vi "unregisterSubscriber.vi"(1 "Parameters":T2) -> (2 "Error out":errorcluster, 3 "Reply":T1, 4 "Reply":string, 5 "registerSubscriber":string)   [LabVIEW 2010]
uses:
  <userlib>/ROSforLV_0.1/ROS/Code/_ROSDefinition.vi
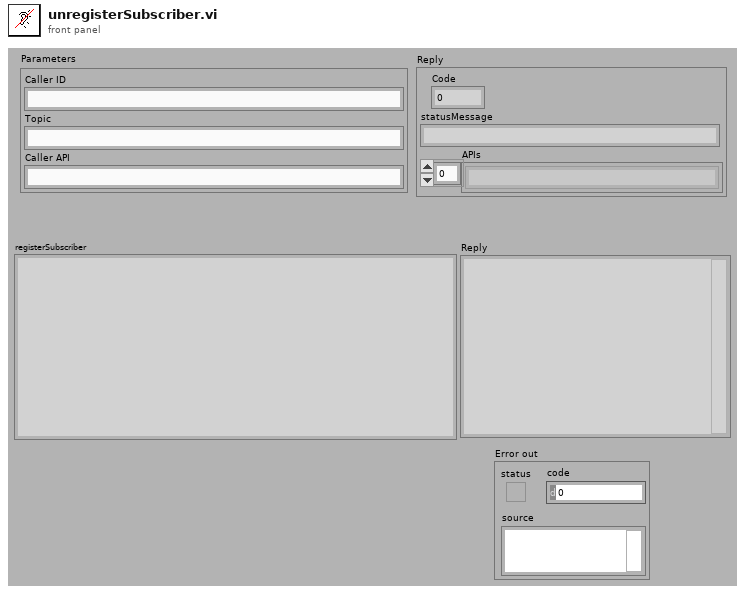
[diagram p1: front panel]
types:
  T1 = cluster{"Code":i8, "statusMessage":string, "APIs":string[]}
  T2 = cluster{"Caller ID":string, "Topic":string, "Caller API":string}
  T3 = cluster{"Code":i8, "statusMessage":string, "APIs":string[]}[]
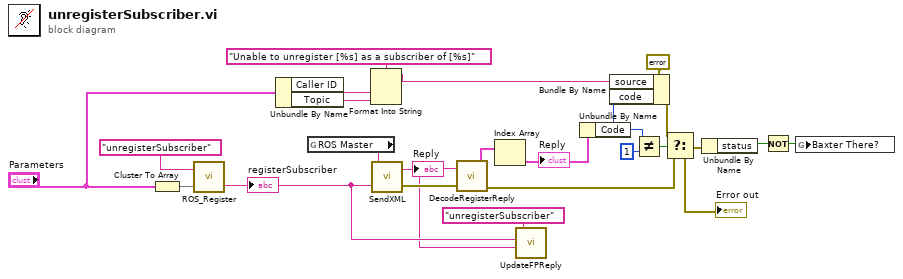
[diagram p0: block diagram]
diagram:
  n1 = Cluster To Array(cluster="Parameters") -> (array=w5:string[])
  n2 = call <userlib>:"ROS_Register.vi"("Parameters"=w5, "Method Name"="unregisterSubscriber") -> ("registerSubscriber"=w3:string)  [unwired: 1 in]
  "registerSubscriber" <- w3
  n3 = Unbundle By Name("Parameters") -> ("Caller ID"=w21:string, "Topic"=w20:string)
  n4 = global read "_ROSDefinition.vi" "ROS Master"() -> (w23:string)
  n5 = Format Into String(format string="Unable to unregister [%s] as a subscriber of [%s]" ("source"), w21, w20) -> (resulting string=w8:string)  [unwired: 2 in, 1 out]
  n6 = call <userlib>:"SendXML.vi"("Send"=w3, "URI in"=w23) -> ("error out"=w9:errorcluster, "Reply"=w2:string)
  "Reply" <- w2
  n7 = call <userlib>:"DecodeRegisterReply.vi"("error in (no error)"=w9, "Response"=w2) -> ("error out"=w13:errorcluster, "Reply"=w17:T3)
  n8 = Index Array(array=w17) -> (element=w16:T1)  [unwired: 1 in]
  "Reply" <- w16
  n9 = call <userlib>:"UpdateFPReply.vi"("Reply"=w2, "Sent"=w3, "method"="unregisterSubscriber" ("name (unnamed)")) -> ()  [unwired: 3 in]
  n10 = Unbundle By Name(w16) -> ("Code"=w12:i8)
  n11 = Bundle By Name(cluster=errorcluster {"status"=TRUE, "code"=0, "source"=" Error"} ("t"), "source"=w8, "code"=w12) -> (w11:errorcluster)
  n12 = Not Equal?(x=w12, y=i8 1) -> (x != y?=w14:bool)
  n13 = Select(t=w11, s=w14, f=w13) -> (s? t:f=w10:errorcluster)
  "Error out" <- w10
  n14 = Unbundle By Name(w10) -> ("status"=w18:bool)
  n15 = Not(x=w18) -> (.not. x?=w19:bool)
  n16 = global write "_ROSDefinition.vi" "Baxter There?"(w19) -> ()
